vi "DBC Get Msg Quantity.vi"(11 "DBCHandle":u64) -> (3 "function return":i32)   [LabVIEW 2010, in "dbc_parser.lvlib"]
doc: "int WINAPI DBC_GetMsgQuantity(long long DBCHandle);"
uses:
  dbc_parser.lvlib
  USB2XXX/trunk/USB2XXX/USB2XXX/vs2019/Release/USB2XXX.dll
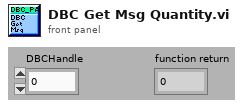
[diagram p1: front panel]
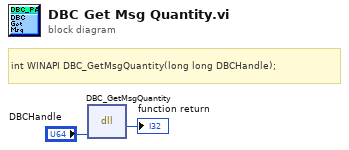
[diagram p0: block diagram]
diagram:
  # "int WINAPI DBC_GetMsgQuantity(long long DBCHandle);"
  n1 = dll-call lib="E:/Projects/USB2XXX/trunk/USB2XXX/USB2XXX/vs2019/Release/USB2XXX.*" fn="DBC_GetMsgQuantity"("DBCHandle"="DBCHandle") -> (→"function return":i32)  [unwired: 4 in, 2 out]
